vi "Table generate_0.vi"() -> ()   [LabVIEW 2015]
panel:
  in  "Tab Control":enum32{"Page 1", "Page 2"}(tab)
  out "Array":i32[][](array[numeric])
  # "Table generate"
  # "Pardeep Kumar"
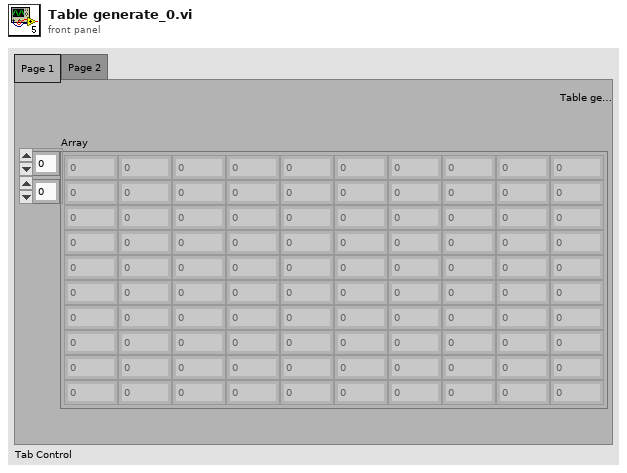
[diagram p1: front panel]
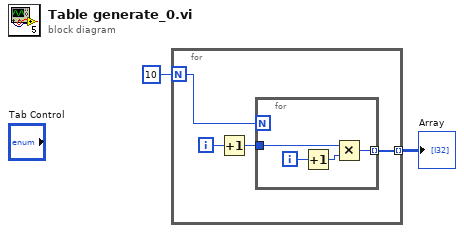
[diagram p0: block diagram]
diagram:
  n1 = for {
    N: 10 -> [w6]
    tunnel: [w3] -> w1 mode=indexing
    i -> [w5]
    n2 = Increment(x=w5) -> (x+1=w4:i32)
    n3 = for {
      N: w6 -> [_]
      tunnel: w4 -> [w9]
      tunnel: [w7] -> w3 mode=indexing
      i -> [w10]
      n4 = Increment(x=w10) -> (x+1=w8:i32)
      n5 = Multiply(x=w9, y=w8) -> (x*y=w7:i32)
    }
  }
  "Array" <- w1
